vi "updateBlinkingSettings.vi"(8 "error in (no error)":errorcluster, 9 "Waveform Duration (s)":dbl=1.0 format="%0.2f", 10 "On and Off time (ms)":u32[](array[numeric])=[500, 500], 11 "LED in":refnum<class "LED.lvclass">) -> (0 "error out":errorcluster, 3 "LED out":refnum<class "LED.lvclass">)   [LabVIEW 2019, in "LED.lvclass"]
uses:
  LED.lvclass
  LED.lvclass/LED.ctl
  Sound/Sound.lvclass
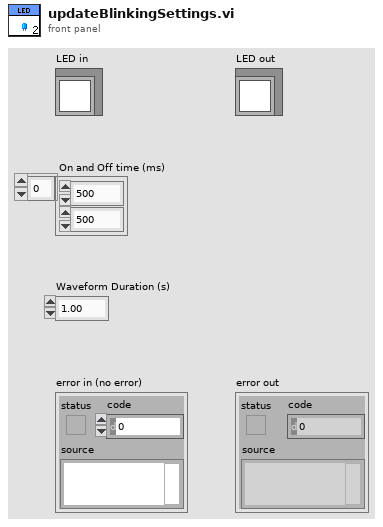
[diagram p1: front panel]
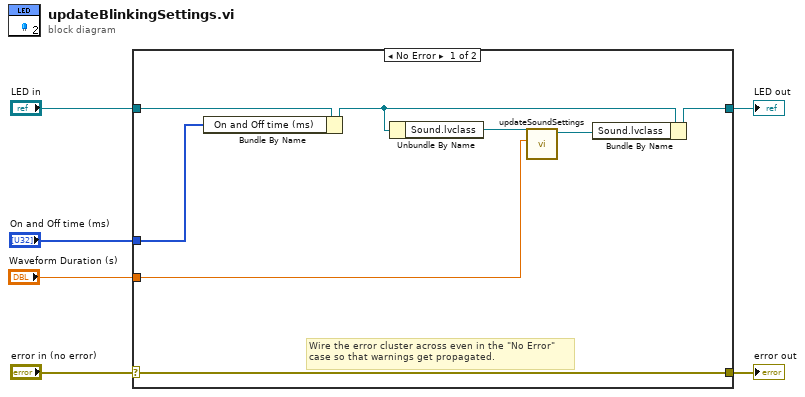
[diagram p0: block diagram]
diagram:
  n1 = case shown="No Error" "error in (no error)" {
    selector: "error in (no error)" -> [w13 w16]
    tunnel: [w13 w16] -> w5
    tunnel: [w10 w15] -> w3
    tunnel: "LED in" -> [w14 w15]
    tunnel: "On and Off time (ms)" -> [w12 _]
    tunnel: "Waveform Duration (s)" -> [w7 _]
    frame No Error {
      # "Wire the error cluster across even in the \"No Error\"\ncase so that warnings get propagated."
      n2 = Bundle By Name(cluster=w14, "On and Off time (ms)"=w12) -> (w11:refnum<class "LED.lvclass">)
      n3 = Unbundle By Name(w11) -> ("Sound.lvclass"=w9:refnum<class "Sound.lvclass">)
      n4 = call "updateSoundSettings.vi"("duration"=w7, "Sound in"=w9) -> ("Sound out"=w8:refnum<class "Sound.lvclass">)  [unwired: 8 in, 1 out]
      n5 = Bundle By Name(cluster=w11, "Sound.lvclass"=w8) -> (w10:refnum<class "LED.lvclass">)
    }
    frame Error {
    }
  }
  "error out" <- w5
  "LED out" <- w3
